vi "Generate Output Files.vi"(4 "Output Folder":path, 5 "Create By-Team CSV":bool, 6 "Create By-Match CSV":bool, 7 "Create schedule.csv":bool, 8 "error in (no error)":errorcluster, 9 "General Data":T1, 10 "Team Info":T2, 11 "Match Array":i32[][](array[numeric])) -> (0 "error out":errorcluster, 2 "By Match List":T3, 3 "By Team List":T3)   [LabVIEW 2013]
uses:
  Team Data Array.ctl
  <vilib>/Utility/file.llb/Write To Spreadsheet File (string).vi
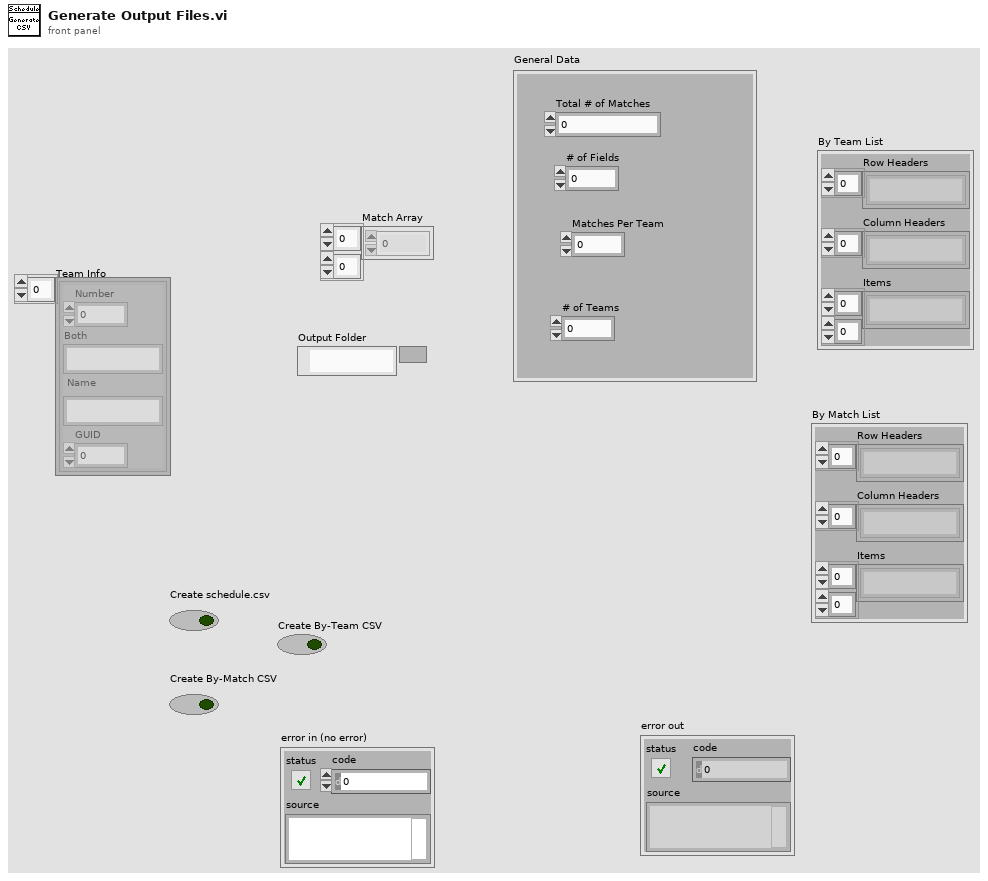
[diagram p1: front panel]
types:
  T1 = cluster{"Total # of Matches":i32, "# of Fields":i32, "Matches Per Team":i32, "# of Teams":i32}
  T2 = typedef "Team Data Array.ctl" = cluster{"Number":u16, "Both":string, "Name":string, "GUID":u16}[]
  T3 = cluster{"Row Headers":string[], "Column Headers":string[], "Items":string[][]}
  T4 = cluster{"Number":u16, "Both":string, "Name":string, "GUID":u16}
  T5 = cluster{"Number":u16, "Name":string, cluster{"Match":i32, "Position":i32}[]}
  T6 = cluster{"Number":u16, "Name":string, cluster{"Match":i32, "Position":i32}[]}[]
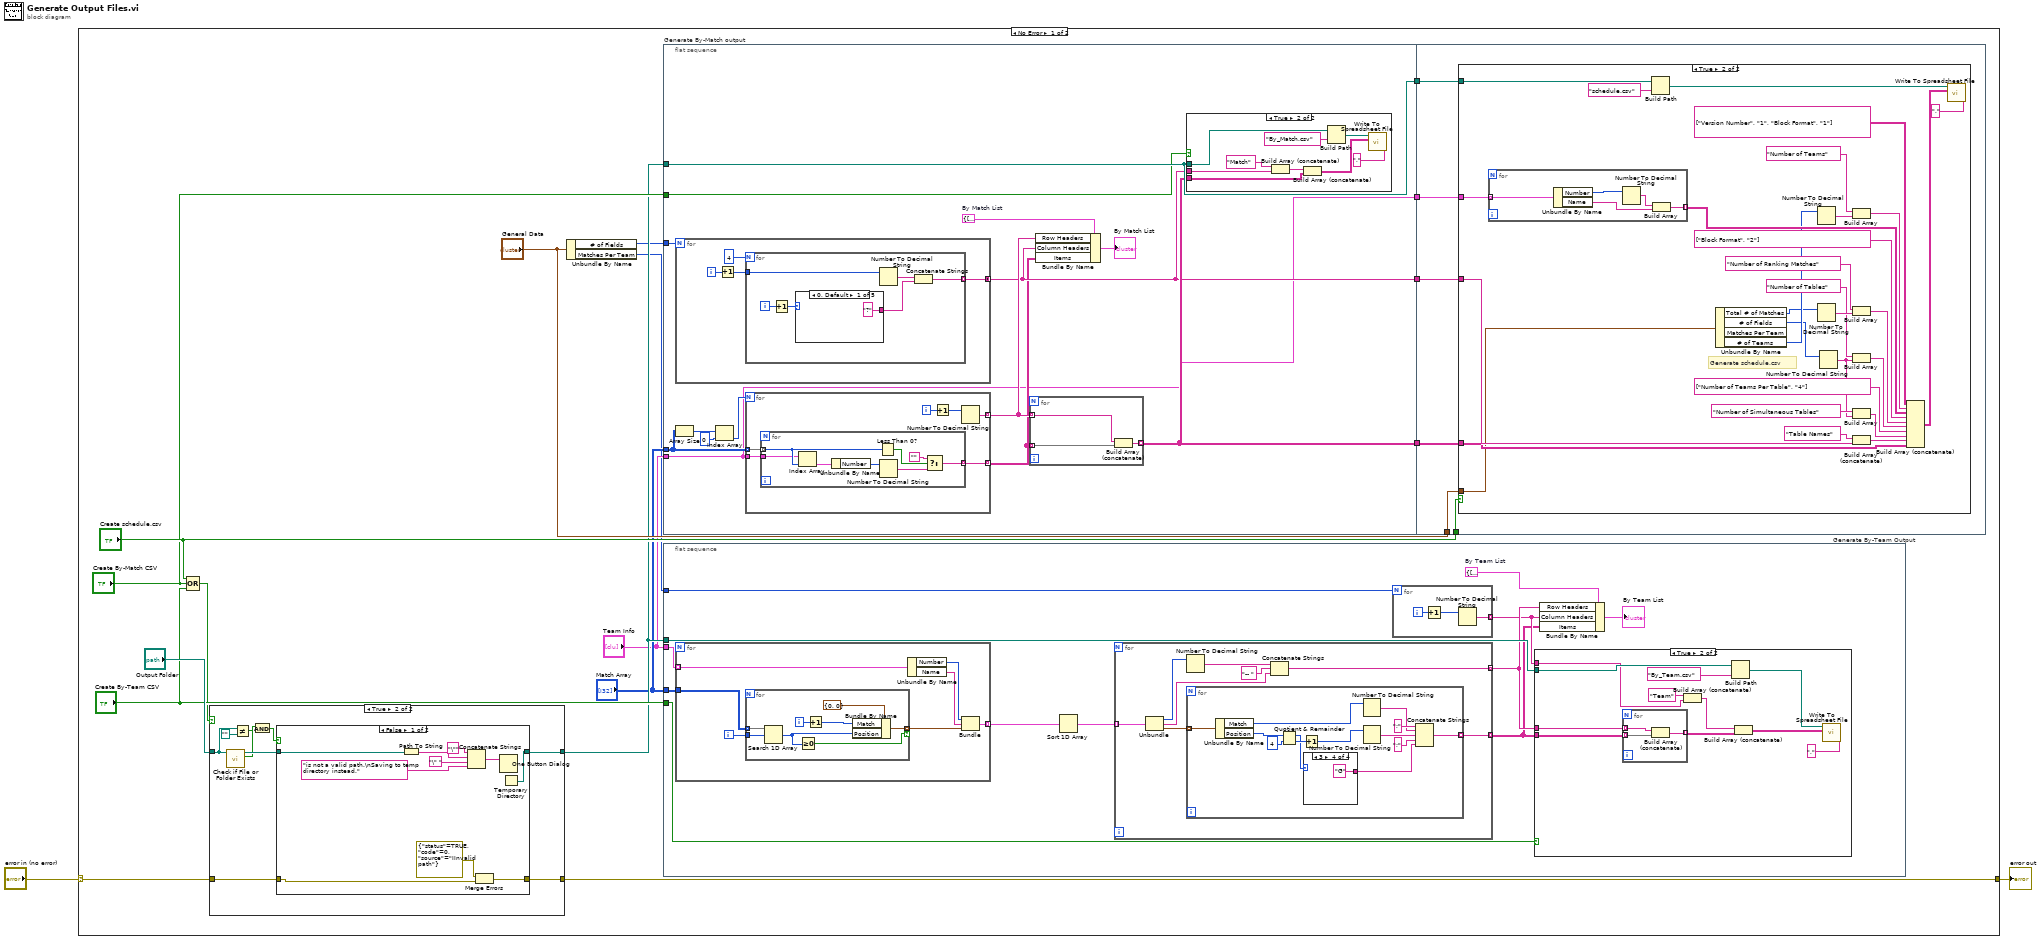
[diagram p0: block diagram]
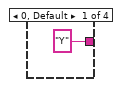
[diagram p5: hidden frame]
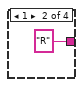
[diagram p6: hidden frame]
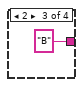
[diagram p7: hidden frame]
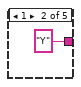
[diagram p9: hidden frame]
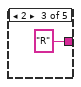
[diagram p10: hidden frame]
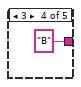
[diagram p11: hidden frame]
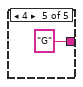
[diagram p12: hidden frame]
diagram:
  n1 = case shown="No Error" "error in (no error)" {
    selector: "error in (no error)" -> [w13 w207]
    tunnel: [w14 w207] -> w2
    frame No Error {
      n2 = Compound Arithmetic op=OR("Create schedule.csv", "Create By-Match CSV", "Create By-Team CSV") -> (w3:bool)
      n3 = case shown="True" w3 {
        tunnel: "Output Folder" -> [w21 w25]
        tunnel: [w20 w30] -> w14
        tunnel: w13 -> [w20 w29]
        tunnel: [w21 w28] -> w8
        frame False {
        }
        frame True {
          n4 = call <vilib>:"Check if File or Folder Exists.vi"("path"=w25) -> ("file or folder exists?"=w24:bool, "dup path"=w27:path)  [unwired: 8 in, 1 out]
          n5 = Not Equal?(x=w25, y=path "") -> (x != y?=w23:bool)
          n6 = And(x=w24, y=w23) -> (x .and. y?=w22:bool)
          n7 = case shown="False" w22 {
            tunnel: w27 -> [w38 w42]
            tunnel: [w40 w42] -> w28
            tunnel: w29 -> [w33 w41]
            tunnel: [w31 w41] -> w30
            frame False {
              n8 = Path To String(path=w38) -> (string=w37:string)
              n9 = Concatenate Strings("\"" ("string"), w37, "\" " ("string"), "is not a valid path.\nSaving to temp directory instead." ("string")) -> (w34:string)
              n10 = Merge Errors(errorcluster {"status"=TRUE, "code"=0, "source"="IInvalid path"} ("error in"), w33) -> (w31:errorcluster)
              n11 = One Button Dialog(message=w34) -> ()  [unwired: 1 in, 1 out]
              n12 = Temporary Directory() -> (w40:path)
            }
            frame True {
            }
          }
        }
      }
      n13 = Unbundle By Name("General Data") -> ("# of Fields"=w5:i32, "Matches Per Team"=w4:i32)
      n14 = flat-sequence "Generate By-Match output" {
        tunnel: "Match Array" -> [w122]
        tunnel: w8 -> [w121]
        tunnel: [w121] -> w12
        tunnel: [w117] -> w11
        tunnel: [w120] -> w10
        tunnel: "Team Info" -> [w114]
        tunnel: [w114] -> w9
        tunnel: w5 -> [w113]
        tunnel: "Create By-Match CSV" -> [w112]
        tunnel: w12 -> [w172]
        tunnel: w11 -> [w171]
        tunnel: w10 -> [w170]
        tunnel: w9 -> [w169]
        tunnel: "General Data" -> [w168]
        tunnel: "Create schedule.csv" -> [w167]
        frame #0 {
          w119 = T3 {"Row Headers"=[], "Column Headers"=[], "Items"=[]}  # By Match List
          n15 = for {
            N: w113 -> [_]
            tunnel: [w153] -> w117 mode=concatenating
            i -> [w155]
            n16 = Increment(x=w155) -> (x+1=w154:i32)
            n17 = for {
              N: 4 -> [_]
              tunnel: w154 -> [w161]
              tunnel: [w158] -> w153 mode=indexing
              i -> [w159]
              n18 = Increment(x=w159) -> (x+1=w157:i32)
              n19 = case shown="0, Default" w157 {
                tunnel: ["?" "Y" "R" "B" "G"] -> w156
                frame 0, Default {
                }
                frame 1 {
                }
                frame 2 {
                }
                frame 3 {
                }
                frame 4 {
                }
              }
              n20 = Number To Decimal String(number=w161) -> (decimal integer string=w160:string)  [unwired: 1 in]
              n21 = Concatenate Strings(w160, w156) -> (w158:string)
            }
          }
          n22 = Array Size(array=w122) -> (size(s)=w125:i32[])
          n23 = Index Array(array=w125, index=0) -> (element=w123:i32)
          n24 = for {
            N: w123 -> [_]
            tunnel: w122 -> [w143] mode=indexing
            tunnel: [w142] -> w116 mode=indexing
            tunnel: [w139] -> w118 mode=indexing
            tunnel: w114 -> [w138]
            i -> [w141]
            n25 = for {
              tunnel: w143 -> [w146] mode=indexing
              tunnel: [w149] -> w142 mode=indexing
              tunnel: w138 -> [w144]
              n26 = Index Array(array=w144, index=w146) -> (element=w151:T4)
              n27 = Unbundle By Name(w151) -> ("Number"=w150:u16)
              n28 = Less Than 0?(x=w146) -> (x < 0?=w145:bool)
              n29 = Number To Decimal String(number=w150) -> (decimal integer string=w148:string)  [unwired: 1 in]
              n30 = Select(t="", s=w145, f=w148) -> (s? t:f=w149:string)
            }
            n31 = Increment(x=w141) -> (x+1=w140:i32)
            n32 = Number To Decimal String(number=w140) -> (decimal integer string=w139:string)  [unwired: 1 in]
          }
          n33 = for {
            tunnel: w116 -> [w136] mode=indexing
            tunnel: w118 -> [w137] mode=indexing
            tunnel: [w135] -> w120 mode=indexing
            n34 = Build Array (concatenate)(w137, w136) -> (w135:string[])
          }
          n35 = Bundle By Name(cluster=w119, "Row Headers"=w118, "Column Headers"=w117, "Items"=w116) -> (→"By Match List":T3)
          n36 = case shown="True" w112 {
            tunnel: w121 -> [_ w128]
            tunnel: w117 -> [_ w127]
            tunnel: w120 -> [_ w126]
            frame False {
            }
            frame True {
              n37 = Build Array (concatenate)("Match", w127) -> (w132:string[])
              n38 = Build Array (concatenate)(w132, w126) -> (w134:string[][])
              n39 = Build Path(base path=w128, name or relative path="By_Match.csv") -> (appended path=w129:path)
              n40 = call-poly <vilib>:"Write To Spreadsheet File.vi"("delimiter (\\t)"="," ("delimiter (\\t)"), "2D data"=w134, "file path (dialog if empty)"=w129) -> ()  [unwired: 5 in, 1 out]
            }
          }
        }
        frame #1 {
          n41 = case shown="True" w167 {
            tunnel: w172 -> [_ w196]
            tunnel: w171 -> [_ w182]
            tunnel: w170 -> [_ w179]
            tunnel: w169 -> [_ w177]
            tunnel: w168 -> [_ w176]
            frame False {
            }
            frame True {
              # "Generate schedule.csv"
              n42 = for {
                tunnel: w177 -> [w206] mode=indexing
                tunnel: [w202] -> w197 mode=indexing
                n43 = Unbundle By Name(w206) -> ("Number"=w205:u16, "Name"=w203:string)
                n44 = Number To Decimal String(number=w205) -> (decimal integer string=w204:string)  [unwired: 1 in]
                n45 = Build Array(w204, w203) -> (w202:string[])
              }
              n46 = Build Path(base path=w196, name or relative path="schedule.csv") -> (appended path=w194:path)
              n47 = Unbundle By Name(w176) -> ("Total # of Matches"=w174:i32, "# of Fields"=w173:i32, "# of Teams"=w175:i32)  [unwired: 1 out]
              n48 = Number To Decimal String(number=w175) -> (decimal integer string=w199:string)  [unwired: 1 in]
              n49 = Number To Decimal String(number=w174) -> (decimal integer string=w189:string)  [unwired: 1 in]
              n50 = Number To Decimal String(number=w173) -> (decimal integer string=w183:string)  [unwired: 1 in]
              n51 = Build Array("Number of Teams", w199) -> (w198:string[])
              n52 = Build Array("Number of Ranking Matches", w189) -> (w190:string[])
              n53 = Build Array("Number of Tables", w183) -> (w188:string[])
              n54 = Build Array("Number of Simultaneous Tables", w183) -> (w185:string[])
              n55 = Build Array (concatenate)("Table Names", w182) -> (w180:string[])
              n56 = Build Array (concatenate)(string[][] [["Version Number", "1"], ["Block Format", "1"]], w198, w197, string[] ["Block Format", "2"], w190, w188, string[] ["Number of Teams Per Table", "4"], w185, w180, w179) -> (w193:string[][])
              n57 = call-poly <vilib>:"Write To Spreadsheet File.vi"("delimiter (\\t)"="," ("delimiter (\\t)"), "2D data"=w193, "file path (dialog if empty)"=w194) -> ()  [unwired: 5 in, 1 out]
            }
          }
        }
      }
      n58 = flat-sequence "Generate By-Team Output" {
        tunnel: "Match Array" -> [w53]
        tunnel: w8 -> [w51]
        tunnel: "Team Info" -> [w45]
        tunnel: w4 -> [w44]
        tunnel: "Create By-Team CSV" -> [w43]
        frame #0 {
          w50 = T3 {"Row Headers"=[], "Column Headers"=[], "Items"=[]}  # By Team List
          n59 = for {
            tunnel: w45 -> [w103] mode=indexing
            tunnel: [w100] -> w52 mode=indexing
            tunnel: w53 -> [w99]
            i -> [w98]
            n60 = for {
              tunnel: w99 -> [w111] mode=indexing
              tunnel: w98 -> [w110]
              tunnel: [w104] -> w97 mode=indexing if=w109
              i -> [w108]
              n61 = Search 1D Array(1D array=w111, element=w110) -> (index of element=w105:i32)  [unwired: 1 in]
              n62 = Greater Or Equal To 0?(x=w105) -> (x >= 0?=w109:bool)
              n63 = Increment(x=w108) -> (x+1=w106:i32)
              n64 = Bundle By Name(cluster=cluster{"Match":i32, "Position":i32} {"Match"=0, "Position"=0}, "Match"=w106, "Position"=w105) -> (w104:cluster{"Match":i32, "Position":i32})
            }
            n65 = Unbundle By Name(w103) -> ("Number"=w102:u16, "Name"=w101:string)
            n66 = Bundle("Number"=w102, "Name"=w101, w97) -> (w100:T5)  [unwired: 1 in]
          }
          n67 = Sort 1D Array(array=w52) -> (sorted array=w54:T6)
          n68 = for {
            tunnel: w54 -> [w79] mode=indexing
            tunnel: [w74] -> w49 mode=indexing
            tunnel: [w72] -> w47 mode=indexing
            n69 = Unbundle(w79) -> ("Number"=w78:u16, "Name"=w75:string, w73:cluster{"Match":i32, "Position":i32}[])
            n70 = Number To Decimal String(number=w78) -> (decimal integer string=w77:string)  [unwired: 1 in]
            n71 = for {
              tunnel: w73 -> [w92] mode=indexing
              tunnel: [w87] -> w72 mode=indexing
              n72 = Unbundle By Name(w92) -> ("Match"=w91:i32, "Position"=w86:i32)
              n73 = Quotient & Remainder(x=w86, y=4) -> (x-y*floor(x/y)=w82:i32, floor(x/y)=w84:i32)
              n74 = Increment(x=w84) -> (x+1=w83:i32)
              n75 = case shown="3" w82 {
                tunnel: ["Y" "R" "B" "G"] -> w81
                frame 0, Default {
                }
                frame 1 {
                }
                frame 2 {
                }
                frame 3 {
                }
              }
              n76 = Number To Decimal String(number=w91) -> (decimal integer string=w90:string)  [unwired: 1 in]
              n77 = Number To Decimal String(number=w83) -> (decimal integer string=w88:string)  [unwired: 1 in]
              n78 = Concatenate Strings(w90, ";" ("string"), w88, ";" ("string"), w81) -> (w87:string)
            }
            n79 = Concatenate Strings(w77, "-- " ("string"), w75) -> (w74:string)
          }
          n80 = for {
            N: w44 -> [_]
            tunnel: [w71] -> w48 mode=indexing
            i -> [w70]
            n81 = Increment(x=w70) -> (x+1=w69:i32)
            n82 = Number To Decimal String(number=w69) -> (decimal integer string=w71:string)  [unwired: 1 in]
          }
          n83 = case shown="True" w43 {
            tunnel: w51 -> [_ w64]
            tunnel: w49 -> [_ w57]
            tunnel: w48 -> [_ w56]
            tunnel: w47 -> [_ w55]
            frame False {
            }
            frame True {
              n84 = for {
                tunnel: w55 -> [w67] mode=indexing
                tunnel: w57 -> [w68] mode=indexing
                tunnel: [w66] -> w61 mode=indexing
                n85 = Build Array (concatenate)(w68, w67) -> (w66:string[])
              }
              n86 = Build Array (concatenate)("Team", w56) -> (w60:string[])
              n87 = Build Path(base path=w64, name or relative path="By_Team.csv") -> (appended path=w62:path)
              n88 = Build Array (concatenate)(w60, w61) -> (w58:string[][])
              n89 = call-poly <vilib>:"Write To Spreadsheet File.vi"("delimiter (\\t)"="," ("delimiter (\\t)"), "2D data"=w58, "file path (dialog if empty)"=w62) -> ()  [unwired: 5 in, 1 out]
            }
          }
          n90 = Bundle By Name(cluster=w50, "Row Headers"=w49, "Column Headers"=w48, "Items"=w47) -> (→"By Team List":T3)
        }
      }
    }
    frame Error {
    }
  }
  "error out" <- w2
